vi "Board Select.vi"   [LabVIEW 2018]
uses:
  <vilib>/rvi/interface/nirviOpenFPGA/nirviOpenFPGA.xnode
  FPGA Bitfiles/LSDurability_Main.lvbitx
  <vilib>/FPGAPlugInAG/sbRIO-9626/niLvFpga_Open_sbRIO-9626.vi
  Controls/FPGA_Reference.ctl
  FPGA Bitfiles/LS_Durability_FPGA_9627.lvbitx
  <vilib>/FPGAPlugInAG/sbRIO-9627/niLvFpga_Open_sbRIO-9627.vi
  <vilib>/rvi/interface/common/dynamic/niFpgaDynamicAddResources.vi
types:
  T1 = typedef "FPGA_Reference.ctl" = refnum<k20>
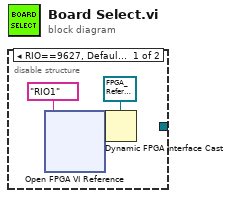
[diagram p0: block diagram]
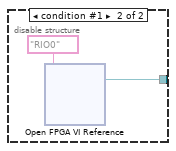
[diagram p2: hidden frame]
diagram:
  n1 = disable-structure shown="RIO==9627, Default" {
    disable-tunnel: [_ w4] -> _
    frame condition #0 (active) {
      n2 = xnode "Open FPGA VI Reference"("resource name"=tag "RIO1") -> ("FPGA VI Reference Out"=w2:refnum<k20>)  [unwired: 1 in, 1 out]
      n3 = Dynamic FPGA Interface Cast(Session In=T1 refnum ("FPGA Interface"), Type=w2) -> ()  [unwired: 1 out]
    }
    frame condition #1 {
      n4 = xnode "Open FPGA VI Reference"("resource name"=tag "RIO0") -> ("FPGA VI Reference Out"=w4:refnum<k20>)  [unwired: 1 in, 1 out]
    }
  }
